vi "Convert_UI_ERD.vi"(0 "New Header?":bool, 2 "ERD Name":string[](array[string]), 5 "ERD_Data_Bundled_Out":T1, 7 "Array":T11[](array[typedef]) {"ERD Number" format="%.0x"}, 11 "Error In":errorcluster) -> (6 "All_ERD_Data_Bundled_Brass":T1, 15 "Error Out":errorcluster)   [LabVIEW 2019]
doc: "This VI parses the data from ERDs in correct format, units, etc. It handles all hex to dec conversions, hex to enum, and hex to boolean conversions.\n\nIf Raw Data from ERD is blank string, then it will output values from shift register."
uses:
  Common/LabVIEW GEA2 Toolkit/GEA3/type defs/ERD Read Data Out.ctl
  type defs/All_Bundled_Data_JL.ctl
  type defs/Version.ctl
  type defs/ERD_Always_Show_JL.ctl
  type defs/CSV_File_String_Arrays.ctl
  type defs/Fault Table Array.ctl
  type defs/Fault_Table_Info.ctl
  type defs/Heat Control.ctl
  type defs/ERD_Commercial_Laundry.ctl
  type defs/BootloaderVersion.ctl
  type defs/ERD_RJ45.ctl
panel:
  out "ERD Number":u16 format="%x"
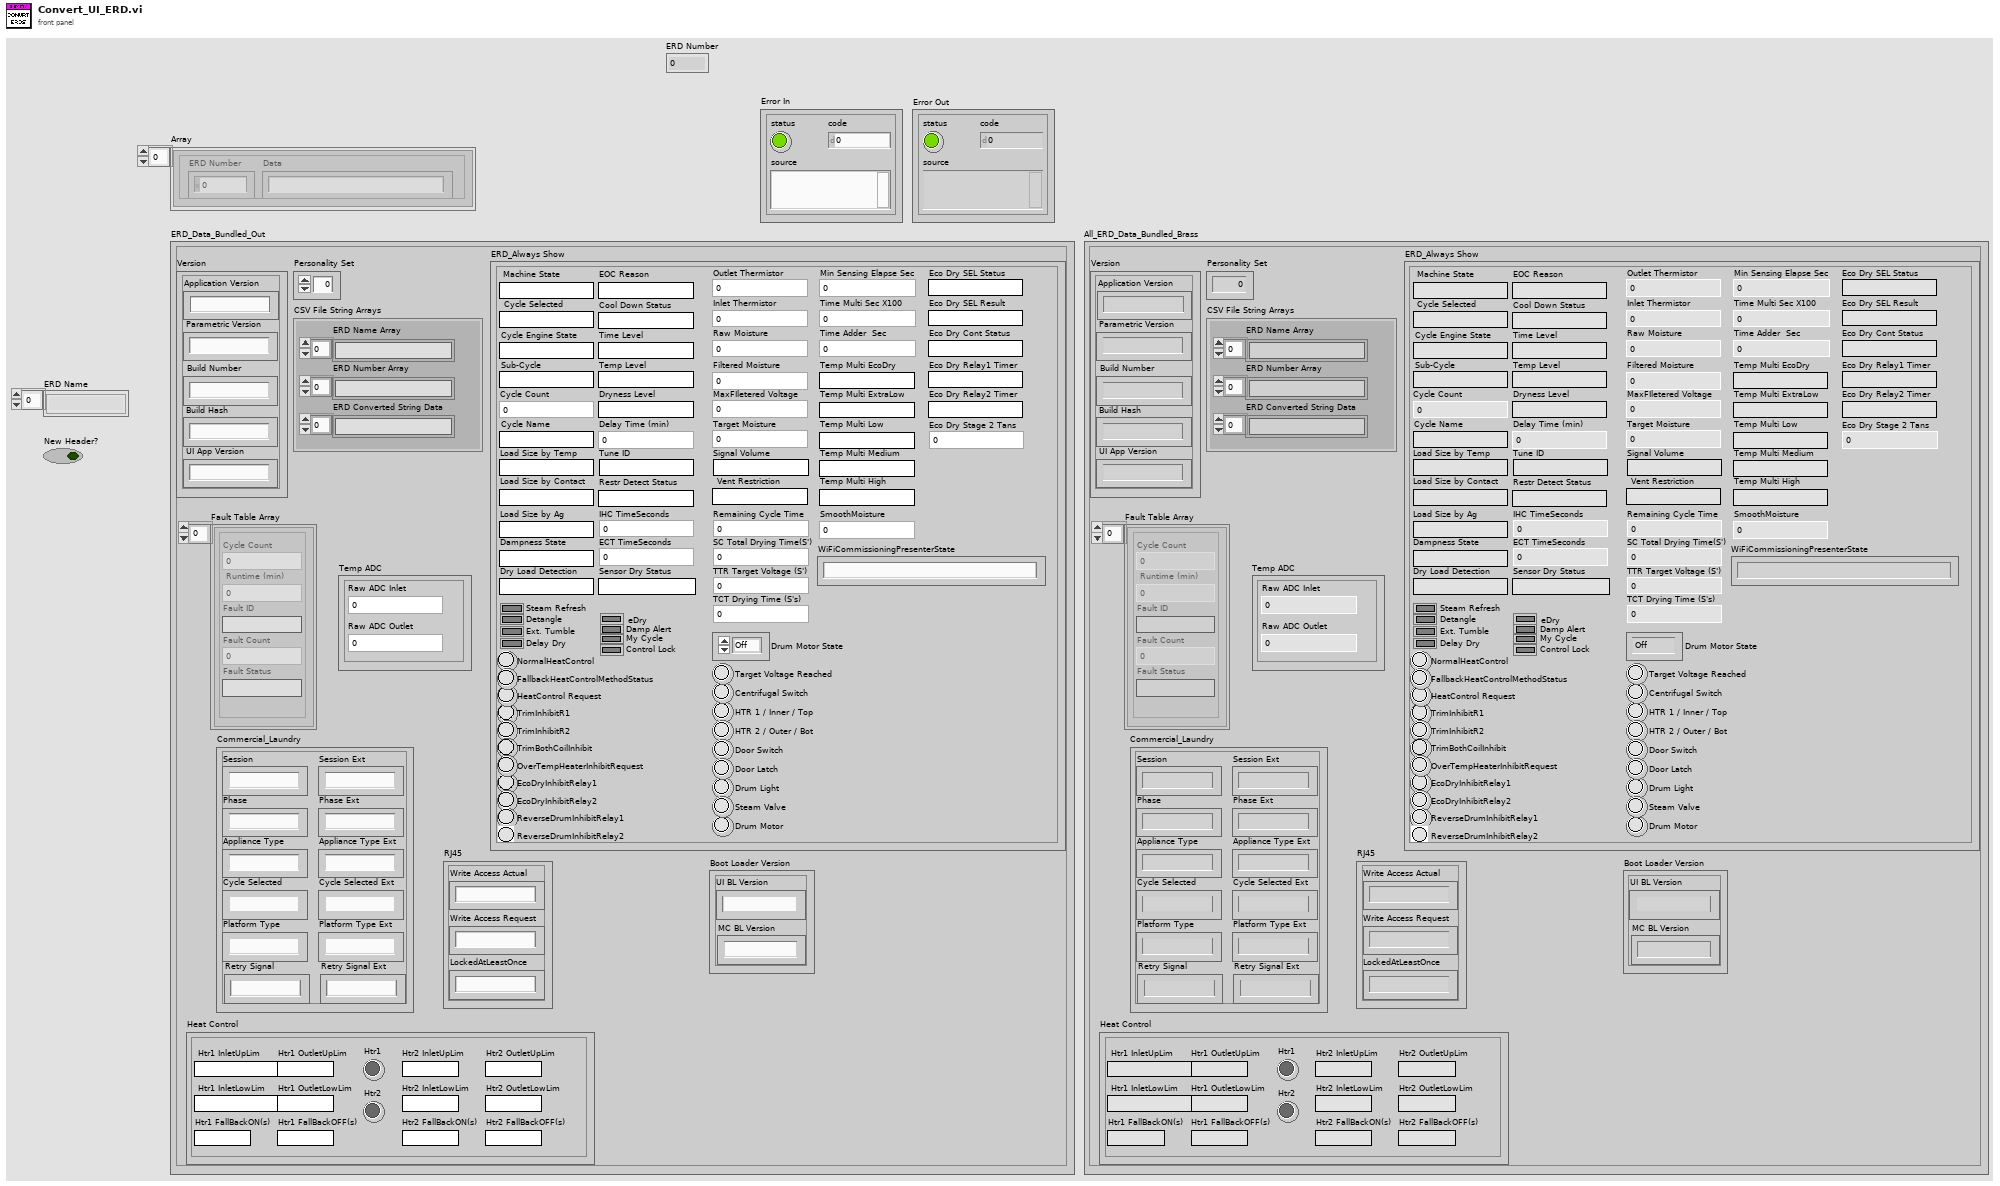
[diagram p1: front panel]
types:
  T1 = typedef "All_Bundled_Data_JL.ctl" = cluster{"Version":T2, "ERD_Always Show":T3, "Personality Set":u8, "CSV File String Arrays":T4, "Fault Table Array ":T5, "Heat Control":T7, "Temp ADC":cluster{"Raw ADC Outlet":u16, "Raw ADC Inlet":u16}, "Commercial_Laundry":T8, "Boot Loader Version":T9, "RJ45":T10}
  T2 = typedef "Version.ctl" = cluster{"Build Number":string, "Build Hash ":string, "Application Version":string, "Parametric Version":string, "UI App Version":string}
  T3 = typedef "ERD_Always_Show_JL.ctl" = cluster{"Inlet Thermistor":u16, "Machine State":string, "Filtered Moisture":u16, "Cycle Selected":string, "HTR 1 / Inner / Top":bool, "HTR 2 / Outer / Bot":bool, "Door Switch":bool, "Drum Light":bool, "Cycle Engine State":string, "Centrifugal Switch":bool, "Drum Motor":bool, "Cycle Count":u32, "Ext. Tumble":bool, "eDry":bool, "Temp Level":string, "Dryness Level":string, "Time Level":string, "Delay Time (min)":u16, "Steam Refresh":bool, "Damp Alert":bool, "Sub-Cycle":string, "Outlet Thermistor":u16, "Target Moisture":u16, "Remaining Cycle Time":u32, "Raw Moisture":u16, "Cycle Name":string, "My Cycle":bool, "Delay Dry":bool, "Detangle":bool, "Control Lock":bool, "Steam Valve":bool, "Door Latch":bool, "Signal Volume":string, "Tune ID":string, "Restr Detect Status":string, "Vent Restriction":string, "Load Size by Contact":string, "Load Size by Temp":string, "EOC Reason":string, "Sensor Dry Status":string, "Dampness State":string, "Target Voltage Reached":bool, "TrimInhibitR1":bool, "TrimInhibitR2":bool, "TrimBothCoilInhibit":bool, "NormalHeatControl":bool, "HeatControl Request":bool, "Cool Down Status":string, "EcoDryInhibitRelay1":bool, "EcoDryInhibitRelay2":bool, "ReverseDrumInhibitRelay1":bool, "ReverseDrumInhibitRelay2":bool, "OverTempHeaterInhibitRequest":bool, "FallbackHeatControlMethodStatus":bool, "IHC TimeSeconds":u32, "ECT TimeSeconds ":u32, "SC Total Drying Time(S')":u32, "TTR Target Voltage (S')":u32, "TCT Drying Time (S's)":u32, "Drum Motor State":enum16{"Off", "Cw", "Ccw", "Max"}, "Load Size by Ag":string, "MaxFIletered Voltage":u16, "Dry Load Detection":string, "Min Sensing Elapse Sec":u32, "Time Multi Sec X100":u32, "Time Adder  Sec":u32, "Temp Multi EcoDry":string, "Temp Multi ExtraLow":string, "Temp Multi Low ":string, "Temp Multi Medium":string, "Temp Multi High":string, "SmoothMoisture":u16, "Eco Dry SEL Status":string, "Eco Dry SEL Result":string, "Eco Dry Cont Status":string, "Eco Dry Relay1 Timer":string, "Eco Dry Relay2 Timer ":string, "Eco Dry Stage 2 Tans ":u32, "WiFiCommissioningPresenterState":string}
  T4 = typedef "CSV_File_String_Arrays.ctl" = cluster{"ERD Number Array":string[], "ERD Name Array":string[], "ERD Converted String Data":string[]}
  T5 = typedef "Fault Table Array.ctl" = T6[]
  T6 = typedef "Fault_Table_Info.ctl" = cluster{"Cycle Count":u32, " Runtime (min) ":u32, "Fault Status":string, "Fault ID":string, "Fault Count":u16}
  T7 = typedef "Heat Control.ctl" = cluster{"Htr1 InletLowLim":string, "Htr1 InletUpLim":string, "Htr1 OutletLowLim":string, "Htr1 OutletUpLim":string, "Htr1 FallBackON(s)":string, "Htr1 FallBackOFF(s)":string, "Htr1":bool, "Htr2 InletLowLim":string, "Htr2 InletUpLim":string, "Htr2 OutletLowLim":string, "Htr2 OutletUpLim":string, "Htr2 FallBackON(s)":string, "Htr2 FallBackOFF(s)":string, "Htr2":bool}
  T8 = typedef "ERD_Commercial_Laundry.ctl" = cluster{"Session":string, "Phase":string, "Appliance Type":string, "Cycle Selected":string, "Platform Type":string, "Retry Signal":string, "Session Ext":string, "Phase Ext":string, "Appliance Type Ext":string, "Cycle Selected Ext":string, "Platform Type Ext":string, "Retry Signal Ext":string}
  T9 = typedef "BootloaderVersion.ctl" = cluster{"UI BL Version":string, "MC BL Version":string}
  T10 = typedef "ERD_RJ45.ctl" = cluster{"Write Access Actual":string, "Write Access Request":string, "LockedAtLeastOnce":string}
  T11 = typedef "ERD Read Data Out.ctl" = cluster{"ERD Number":u16, "Data":string}
  T12 = cluster{"Raw ADC Outlet":u16, "Raw ADC Inlet":u16}
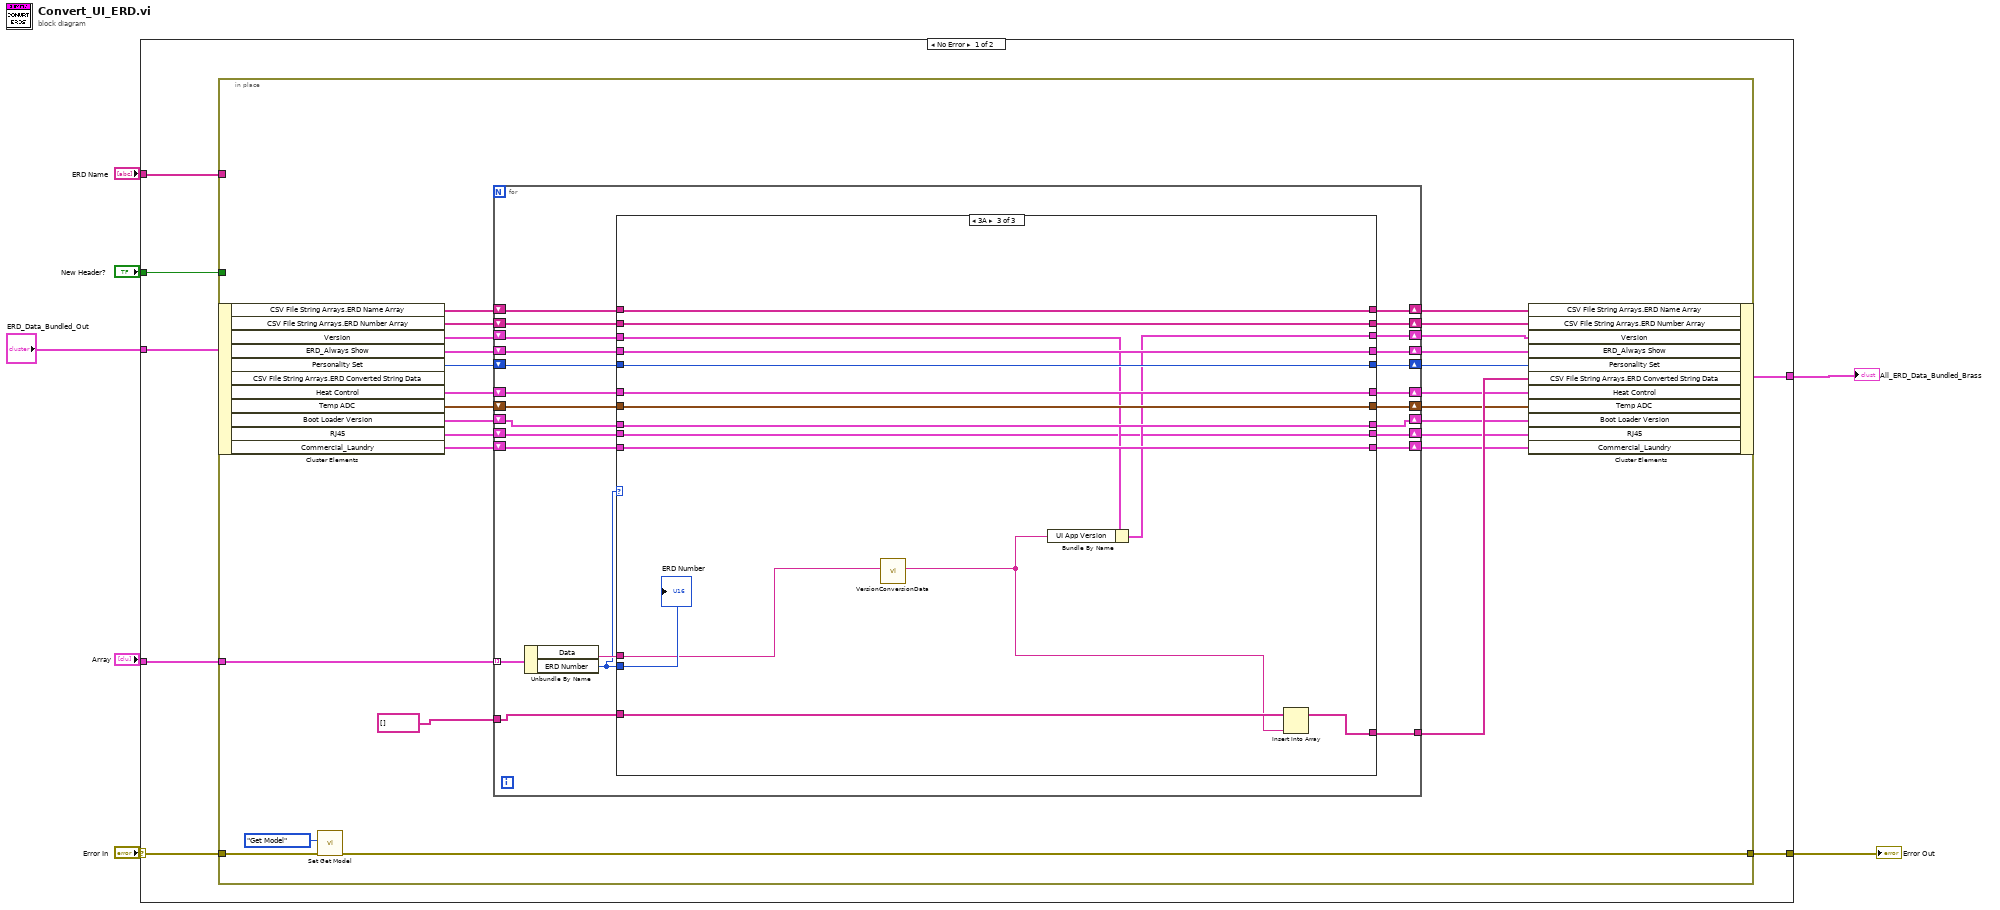
[diagram p0: block diagram]
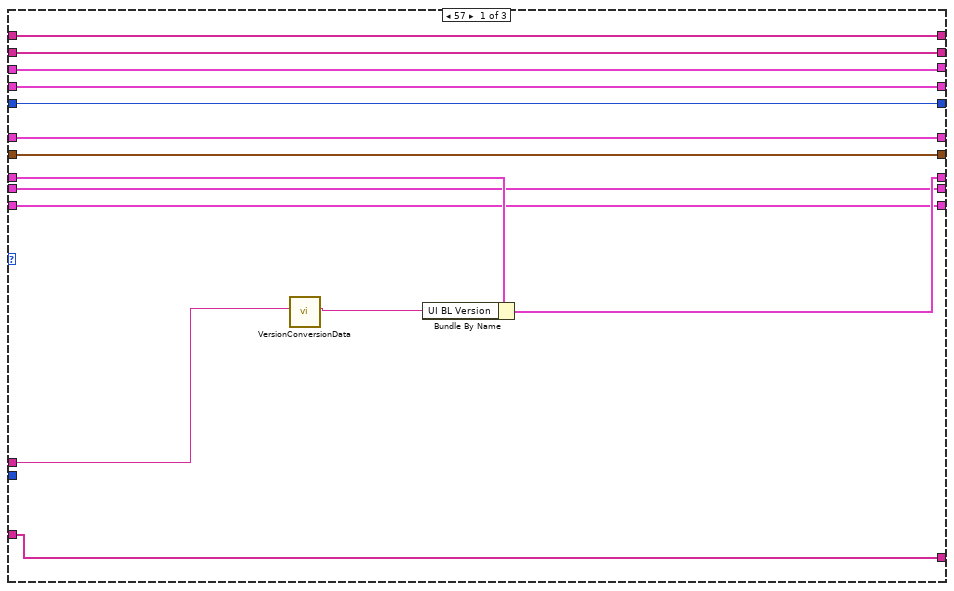
[diagram p2: hidden frame]
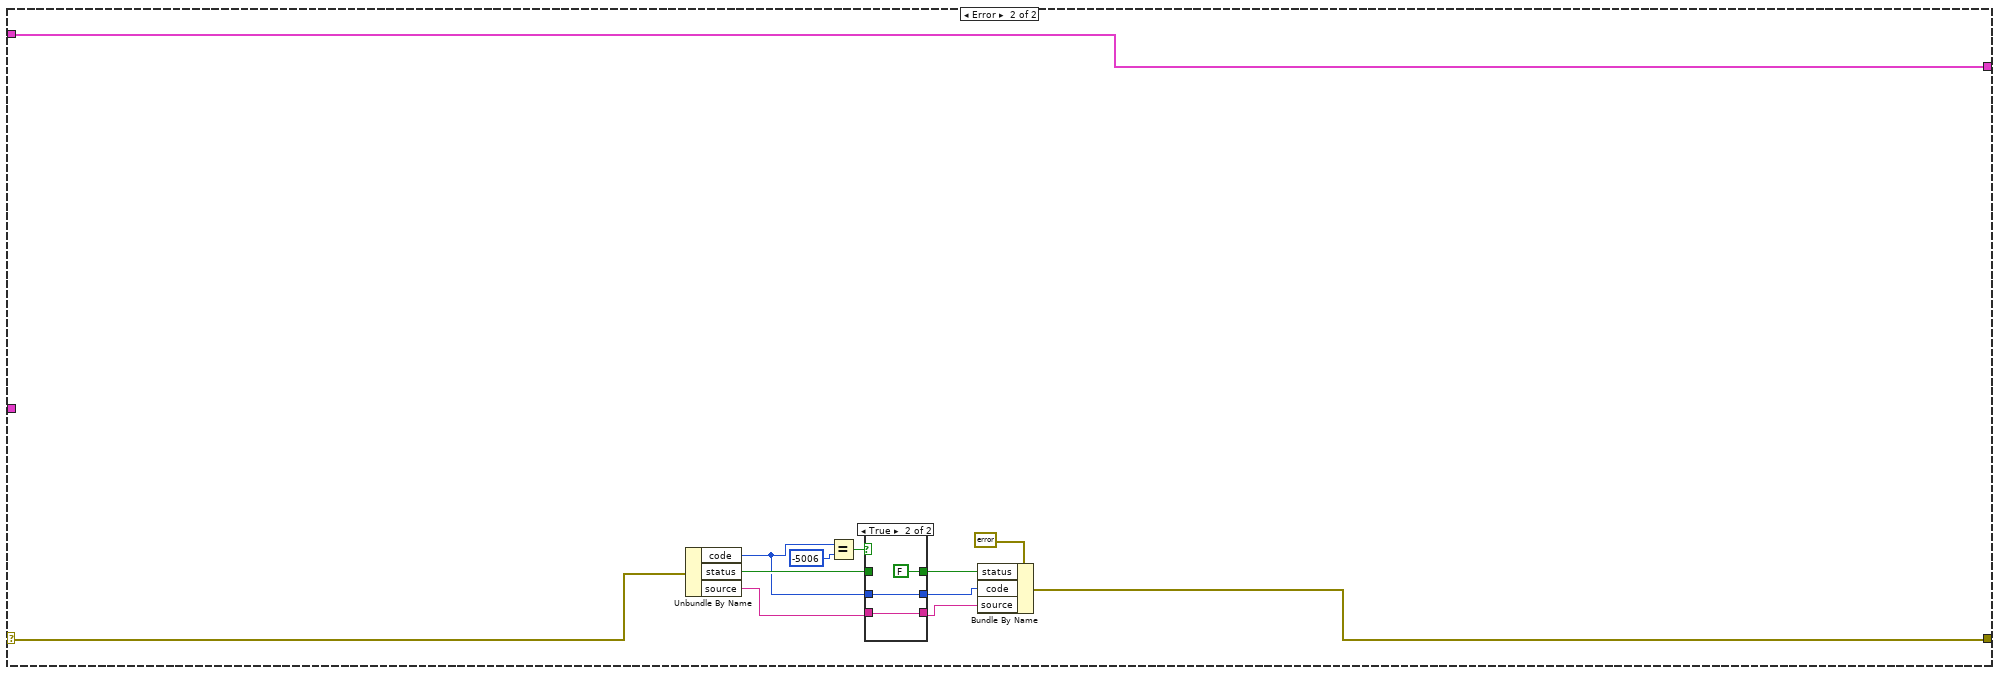
[diagram p4: hidden frame]
diagram:
  n1 = case shown="No Error" "Error In" {
    selector: "Error In" -> [w11 w109]
    tunnel: "Array" -> [w14 _]
    tunnel: [w12 w108] -> w5
    tunnel: "ERD_Data_Bundled_Out" -> [w13 w107]
    tunnel: [w10 w107] -> w4
    tunnel: "New Header?" -> [w9 _]
    tunnel: "ERD Name" -> [w8 _]
    frame No Error {
      n2 = in-place {
        in-place-border: w14 -> [w35]
        in-place-border: [w37] -> w12
        in-place-border: w11 -> [w38]
        in-place-border: w9 -> [_]
        in-place-border: w8 -> [_]
        n3 = in-place-cluster #1(w13) -> ("CSV File String Arrays.ERD Name Array"=w20:string[], "CSV File String Arrays.ERD Number Array"=w19:string[], "Version"=w23:T2, "ERD_Always Show"=w24:T3, "Personality Set"=w26:u8, "Heat Control"=w28:T7, "Temp ADC"=w30:T12, "Boot Loader Version"=w33:T9, "RJ45"=w16:T10, "Commercial_Laundry"=w31:T8)  [unwired: 1 out]
        n4 = call "Set Get Model.vi"("Error In"=w38, "Action"=enum16{"Set Model", "Get Model"}."Get Model") -> ("Error Out"=w37:errorcluster)  [unwired: 8 in, 1 out]
        n5 = for {
          tunnel: string[] [] ("ERD String Data") -> [w62]
          tunnel: [w65] -> w39
          tunnel: w35 -> [w63] mode=indexing
          shift-right: [w59] -> w34
          shift-left: w33 -> [w60]
          shift-right: [w58] -> w32
          shift-left: w31 -> [w57]
          shift-right: [w55] -> w29
          shift-left: w30 -> [w56]
          shift-right: [w53] -> w27
          shift-left: w28 -> [w54]
          shift-right: [w46] -> w21
          shift-left: w20 -> [w45]
          shift-right: [w43] -> w18
          shift-left: w19 -> [w44]
          shift-right: [w47] -> w22
          shift-left: w23 -> [w48]
          shift-right: [w49] -> w17
          shift-left: w24 -> [w50]
          shift-right: [w51] -> w25
          shift-left: w26 -> [w52]
          shift-right: [w41] -> w15
          shift-left: w16 -> [w42]
          n6 = Unbundle By Name(w63) -> ("Data"=w64:string, "ERD Number"=w61:u16)
          n7 = case shown="3A" w61 {
            tunnel: [w79 w89 w106] -> w65
            tunnel: w64 -> [w67 _ w92]
            tunnel: w61 -> [_ _ w105]
            tunnel: w62 -> [w79 w89 w104]
            tunnel: w60 -> [w78 w90 w96]
            tunnel: [w77 w90 w96] -> w59
            tunnel: [w76 w81 w97] -> w58
            tunnel: w57 -> [w76 w81 w97]
            tunnel: w56 -> [w75 w82 w98]
            tunnel: [w75 w82 w98] -> w55
            tunnel: w54 -> [w74 w83 w99]
            tunnel: [w74 w83 w99] -> w53
            tunnel: w52 -> [w73 w84 w100]
            tunnel: [w73 w84 w100] -> w51
            tunnel: w50 -> [w72 w85 w101]
            tunnel: [w72 w85 w101] -> w49
            tunnel: w48 -> [w71 w86 w95]
            tunnel: [w71 w86 w94] -> w47
            tunnel: [w70 w88 w103] -> w46
            tunnel: w45 -> [w70 w88 w103]
            tunnel: w44 -> [w69 w87 w102]
            tunnel: [w69 w87 w102] -> w43
            tunnel: w42 -> [w68 w80 w93]
            tunnel: [w68 w80 w93] -> w41
            frame 57 {
              n8 = call "VersionConversionData.vi"("Version In"=w67) -> ("Version Out"=w66:string)  [unwired: 9 in, 1 out]
              n9 = Bundle By Name(cluster=w78, "UI BL Version"=w66) -> (w77:T9)
            }
            frame 59, Default {
            }
            frame 58 {
              n10 = call "VersionConversionData.vi"("Version In"=w92) -> ("Version Out"=w91:string)  [unwired: 9 in, 1 out]
              n11 = Bundle By Name(cluster=w95, "UI App Version"=w91) -> (w94:T2)
              n12 = Insert Into Array(array=w104, new element=w91) -> (w106:string[])  [unwired: 1 in]
              "ERD Number" <- w105
            }
          }
        }
        n13 = in-place-cluster #1("CSV File String Arrays.ERD Name Array"=w21, "CSV File String Arrays.ERD Number Array"=w18, "Version"=w22, "ERD_Always Show"=w17, "Personality Set"=w25, "CSV File String Arrays.ERD Converted String Data"=w39, "Heat Control"=w27, "Temp ADC"=w29, "Boot Loader Version"=w34, "RJ45"=w15, "Commercial_Laundry"=w32) -> (w10:T1)
      }
    }
    frame Error {
      n14 = Unbundle By Name(w109) -> ("code"=w113:i32, "status"=w114:bool, "source"=w111:string)
      n15 = Equal?(x=w113, y=-5006) -> (x = y?=w117:bool)
      n16 = case shown="True" w117 {
        tunnel: [w121 FALSE] -> w115
        tunnel: w114 -> [w121 _]
        tunnel: w113 -> [w120 w123]
        tunnel: [w120 w123] -> w112
        tunnel: [w119 w122] -> w110
        tunnel: w111 -> [w119 w122]
        frame False {
        }
        frame True {
        }
      }
      n17 = Bundle By Name(cluster=errorcluster {"status"=FALSE, "code"=0, "source"=""} ("error constant"), "status"=w115, "code"=w112, "source"=w110) -> (w108:errorcluster)
    }
  }
  "Error Out" <- w5
  "All_ERD_Data_Bundled_Brass" <- w4
